vi "Write Protocol ID.vi"(10 "Protocol ID":u16, 11 "IP Data Unit in":refnum<class "IP Data Unit.lvclass">) -> (3 "IP Data Unit out":refnum<class "IP Data Unit.lvclass">)   [LabVIEW 2013, in "IP Data Unit.lvclass"]
uses:
  IP Data Unit.lvclass
  IP Data Unit.lvclass/IP Data Unit.ctl
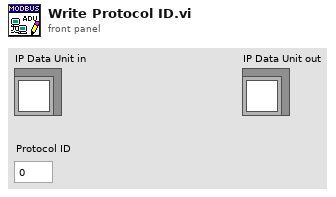
[diagram p1: front panel]
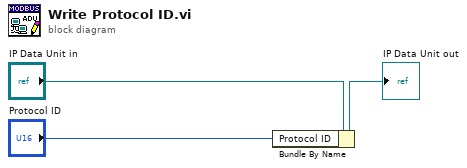
[diagram p0: block diagram]
diagram:
  n1 = Bundle By Name(cluster="IP Data Unit in", "Protocol ID"="Protocol ID") -> (→"IP Data Unit out":refnum<class "IP Data Unit.lvclass">)
